vi "Lower.vi"(8 "error in (no error)":errorcluster, 10 "Speed":dbl=-0.75 format="%#_13g", 11 "Gantry In":refnum<k24>) -> (0 "error out":errorcluster, 3 "Gantry Out":refnum<k24>)   [LabVIEW 2021, in "A3200.lvclass"]
uses:
  A3200.lvclass
  C:/Program Files (x86)/Aerotech/A3200/LabVIEW/2010/Bin/Aerotech.A3200.dll
  Program Files (x86)/Aerotech/A3200/LabVIEW/2010/Bin/Aerotech.A3200.dll
  Drivers/Aerotech A3200/Motion/FreerunSingle.vi
  A3200.lvclass/A3200.ctl
  Drivers/Aerotech A3200/Aerotech.lvlib
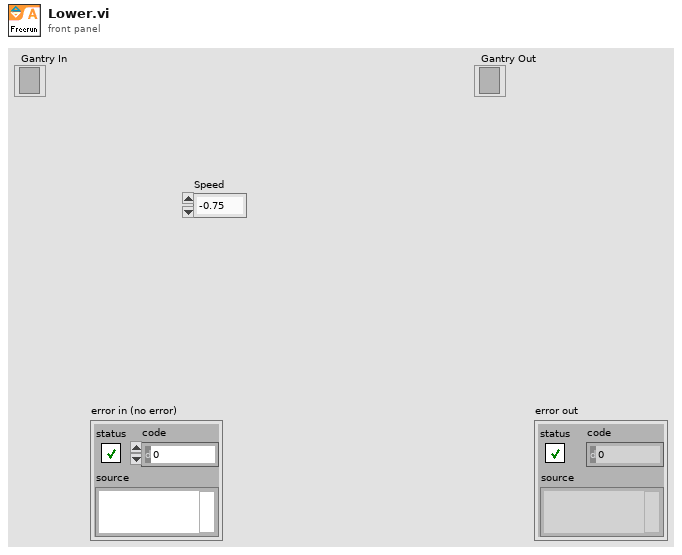
[diagram p1: front panel]
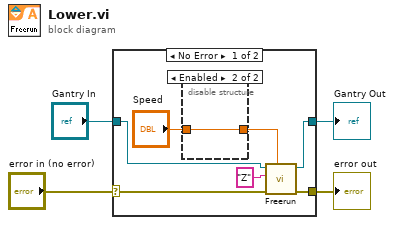
[diagram p0: block diagram]
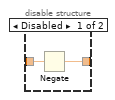
[diagram p2: hidden frame]
diagram:
  n1 = case shown="No Error" "error in (no error)" {
    selector: "error in (no error)" -> [w11 w16]
    tunnel: [w10 w16] -> w3
    tunnel: "Gantry In" -> [w6 w15]
    tunnel: [w5 w15] -> w1
    frame No Error {
      n2 = disable-structure shown="Enabled" {
        disable-tunnel: "Speed" -> [w13 w14]
        disable-tunnel: [w12 w14] -> w7
        frame Disabled {
          n3 = Negate(x=w13) -> (-x=w12:dbl)
        }
        frame Enabled {
        }
      }
      n4 = call-poly "Freerun.vi"("speed"=w7, "error in (no error)"=w11, "axis name"="Z", "controller in"=w6) -> ("error out"=w10:errorcluster, "controller out"=w5:refnum<k24>)  [unwired: 6 in]
    }
    frame Error {
    }
  }
  "error out" <- w3
  "Gantry Out" <- w1
